vi "Send RDS Message Over LSR.vi"(8 "error in (no error)":errorcluster, 10 "RDS Child Message":refnum<class "RDS Message.lvclass">, 11 "LSR Instrument in":refnum<class "LSR Instrument.lvclass">) -> (0 "error out":errorcluster, 3 "LSR Instrument out":refnum<class "LSR Instrument.lvclass">)   [LabVIEW 2015, in "LSR Instrument.lvlib" / "LSR Instrument.lvclass"]
uses:
  LSR Instrument.lvclass
  LSR Transmission/LSR Transmission.lvlib
  Libraries/RDS Serial Handler/RDS Serial Frame.lvclass
  Actors/RDS Serial Instrument Actor/RDS Serial Instrument Actor.lvclass
  Libraries/RDS Framework/RDS Message Class/RDS Message.lvclass
panel:
  out "length":i32
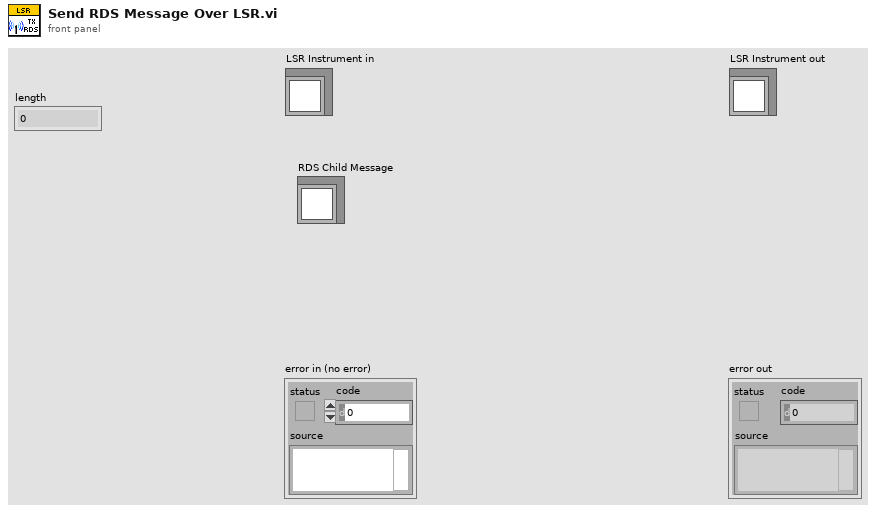
[diagram p1: front panel]
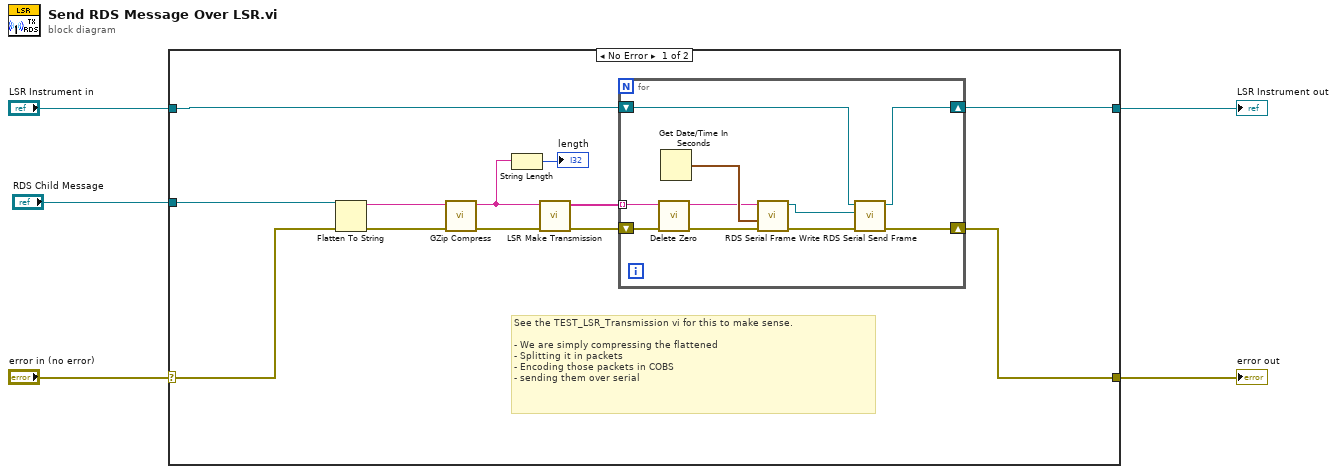
[diagram p0: block diagram]
diagram:
  n1 = case shown="No Error" "error in (no error)" {
    selector: "error in (no error)" -> [w12 w29]
    tunnel: [w14 w29] -> w4
    tunnel: [w15 w28] -> w5
    tunnel: "LSR Instrument in" -> [w13 w28]
    tunnel: "RDS Child Message" -> [w10 _]
    frame No Error {
      # "See the TEST_LSR_Transmission vi for this to make sense. \n\n- We are simply compressing the flattened \n- Splitting it in packets \n- Encoding those packets in COBS\n- sending them over serial"
      n2 = Flatten To String(anything=w10, error in (no error)=w12) -> (data string=w16:string, error out=w11:errorcluster)  [unwired: 2 in, 1 out]
      n3 = call "GZip Compress.vi"("error in (no error)"=w11, "Uncompressed string"=w16) -> ("error out"=w6:errorcluster, "GZip compressed string"=w9:string)  [unwired: 7 in, 1 out]
      n4 = String Length(string=w9) -> (length=→"length":i32)
      n5 = call "LSR Make Transmission.vi"("error in (no error)"=w6, "Data String"=w9) -> ("error out"=w7:errorcluster, "Transmission"=w8:string[])  [unwired: 8 in]
      n6 = for {
        tunnel: w8 -> [w27] mode=indexing
        shift-right: [w20] -> w14
        shift-left: w7 -> [w26]
        shift-right: [w18] -> w15
        shift-left: w13 -> [w19]
        n7 = call "Delete Zero.vi"("error in (no error)"=w26, "COBS String in"=w27) -> ("error out"=w23:errorcluster, "String out"=w24:string)  [unwired: 8 in]
        n8 = Get Date/Time In Seconds() -> (seconds since 1Jan1904=w25:timestamp)
        n9 = call "RDS Serial Frame Write.vi"("error in (no error)"=w23, "Time Stamp"=w25, "Serial String"=w24) -> ("error out"=w21:errorcluster, "RDS Serial Frame out"=w22:refnum<class "RDS Serial Frame.lvclass">)  [unwired: 7 in]
        n10 = call "RDS Serial Send Frame.vi"("error in (no error)"=w21, "RDS Frame"=w22, "RDS Serial Instrument Actor in"=w19) -> ("error out"=w20:errorcluster, "RDS Serial Instrument Actor out"=w18:refnum<class "LSR Instrument.lvclass">)  [unwired: 7 in]
      }
    }
    frame Error {
    }
  }
  "error out" <- w4
  "LSR Instrument out" <- w5
